vi "Get Method Name.vi"(11 "Message Maker in":refnum<class "Message Scripter.lvclass">) -> (2 "Method Name":string)   [LabVIEW 2020, in "Message Maker.lvlib" / "Message Scripter.lvclass"]
uses:
  Message Scripter.lvclass
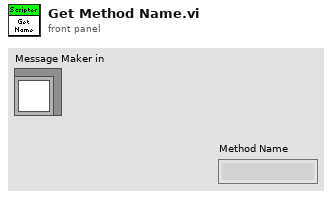
[diagram p1: front panel]
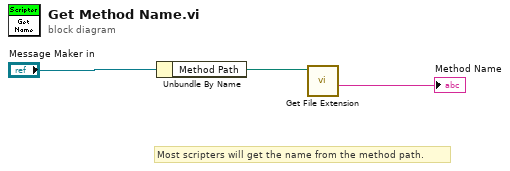
[diagram p0: block diagram]
diagram:
  # "Most scripters will get the name from the method path."
  n1 = Unbundle By Name("Message Maker in") -> ("Method Path"=w2:path)
  n2 = call <vilib>:"Get File Extension.vi"("file"=w2) -> ("filename without extension"=→"Method Name":string)  [unwired: 6 in, 4 out]
